vi "Read OS Name.vi"(8 "error in (no error)":errorcluster, 11 "Board in":refnum<class "Board.lvclass">) -> (0 "error out":errorcluster, 2 "OS Name":string, 3 "Board out":refnum<class "Board.lvclass">)   [LabVIEW 2025, in "Board.lvclass"]
uses:
  Board.lvclass
  Board.lvclass/Board.ctl
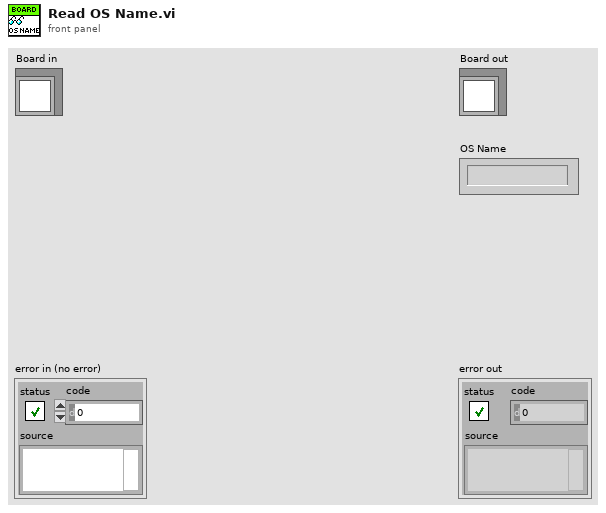
[diagram p1: front panel]
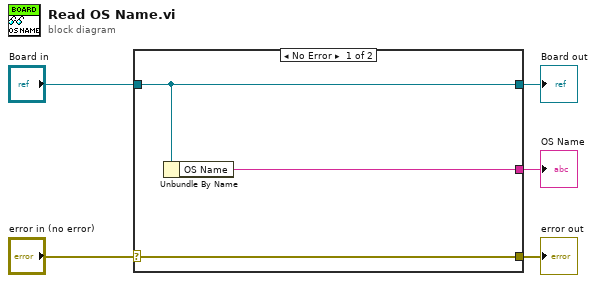
[diagram p0: block diagram]
diagram:
  n1 = case shown="No Error" "error in (no error)" {
    selector: "error in (no error)" -> [w8 w9]
    tunnel: [w8 w9] -> w4
    tunnel: [w7 w10] -> w2
    tunnel: "Board in" -> [w7 w10]
    tunnel: [w6 _] -> w1
    frame No Error {
      n2 = Unbundle By Name(w7) -> ("OS Name"=w6:string)
    }
    frame Error {
    }
  }
  "error out" <- w4
  "Board out" <- w2
  "OS Name" <- w1
